vi "UTIL Predict Class with Variance.vi"(4 "Cluster Data From File":dbl[][](array[numeric]), 5 "Data Point":dbl[](array[numeric])) -> (1 "Sleep Stage":i32)   [LabVIEW 2010]
doc: "This VI approximates the current sleep state given a data point. It uses an approximation of conditional probability, the variance normalized distance from a cluster centroid multiplied by the state porbabilities, and assigns the class of maximum probability.\n\nInputs:\n Data Point 1D Array of DBL, Current data point\n in 3D feature space\n Cluster Data From File 2D Array of DBL,MATLAB computed \n centroids and variances of clusters\n\n\nOutputs:\n Sleep Stage SGL, assigned sleep stage prediction"
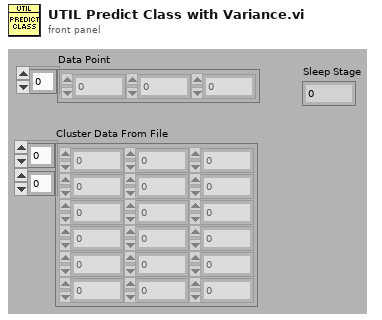
[diagram p1: front panel]
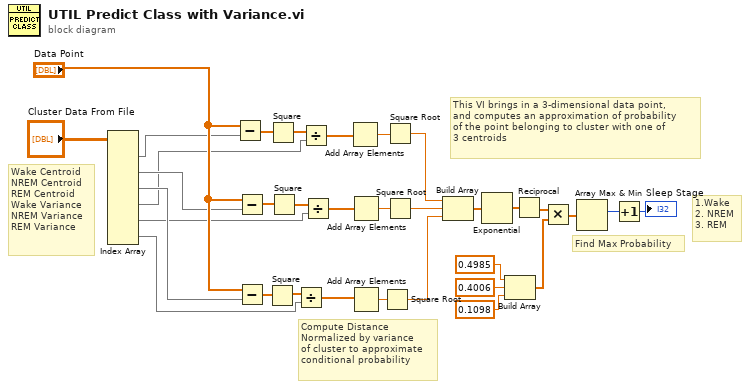
[diagram p0: block diagram]
diagram:
  # "Wake Centroid\nNREM Centroid\nREM Centroid\nWake Variance\nNREM Variance\nREM Variance"
  # "This VI brings in a 3-dimensional data point,\nand computes an approximation of probability\nof the point belonging to cluster with one of \n3 centroids"
  # "1.Wake\n2. NREM\n3. REM"
  # "Find Max Probability"
  # "Compute Distance\nNormalized by variance \nof cluster to approximate \nconditional probability"
  n1 = Index Array(array="Cluster Data From File") -> (element #1=w22:dbl[], element #2=w20:dbl[], element #3=w19:dbl[], element #4=w8:dbl[], element #5=w12:dbl[], element #6=w16:dbl[])  [unwired: 12 in]
  n2 = Subtract(x="Data Point", y=w22) -> (x-y=w10:dbl[])
  n3 = Subtract(x="Data Point", y=w20) -> (x-y=w14:dbl[])
  n4 = Subtract(x="Data Point", y=w19) -> (x-y=w18:dbl[])
  n5 = Square(x=w18) -> (x^2=w17:dbl[])
  n6 = Square(x=w10) -> (x^2=w9:dbl[])
  n7 = Square(x=w14) -> (x^2=w13:dbl[])
  n8 = Divide(x=w17, y=w16) -> (x/y=w15:dbl[])
  n9 = Divide(x=w9, y=w8) -> (x/y=w7:dbl[])
  n10 = Divide(x=w13, y=w12) -> (x/y=w11:dbl[])
  n11 = Add Array Elements(numeric array=w7) -> (sum=w27:dbl)
  n12 = Add Array Elements(numeric array=w11) -> (sum=w28:dbl)
  n13 = Add Array Elements(numeric array=w15) -> (sum=w29:dbl)
  n14 = Square Root(x=w29) -> (sqrt(x)=w32:dbl)
  n15 = Square Root(x=w27) -> (sqrt(x)=w31:dbl)
  n16 = Square Root(x=w28) -> (sqrt(x)=w30:dbl)
  n17 = Build Array(w31, w30, w32) -> (w25:dbl[])
  n18 = Exponential(1:w25) -> (0:w24:dbl[])
  n19 = Build Array(0.4985, 0.4006, 0.1098) -> (w2:dbl[])
  n20 = Reciprocal(x=w24) -> (1/x=w6:dbl[])
  n21 = Multiply(x=w6, y=w2) -> (x*y=w1:dbl[])
  n22 = Array Max & Min(array=w1) -> (max index (indices)=w23:i32)  [unwired: 3 out]
  n23 = Increment(x=w23) -> (x+1=→"Sleep Stage":i32)
